vi "real64_divide.vi"(10 "denominator":dbl, 11 "numerator":dbl) -> (3 "quotient":dbl)   [LabVIEW 2020]
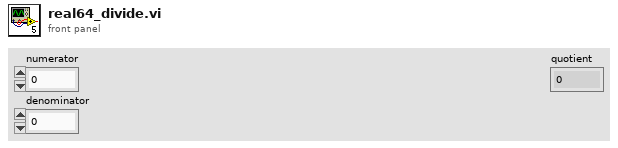
[diagram p1: front panel]
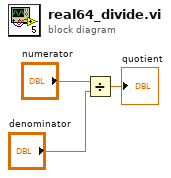
[diagram p0: block diagram]
diagram:
  n1 = Divide(x="numerator", y="denominator") -> (x/y=→"quotient":dbl)
